vi "CRYUnflatten Post Processing.vi"(11 "Unflatten Post Processing":string) -> (0 "Error?":bool, 2 "Post-Processing":T1 {"user equation cluster"."Results axis" items=["x", "y", "z"]; "user equation cluster"."Input axis" items=["x", "y", "z"]; "user equation cluster"."Custom unit results array"."dB ref" format="%.2f"; "user equation cluster"."Custom unit input array"."dB ref" format="%.2f"; "Constant" format="%#.5p"; "Unary Operator" format="%10.0f"; "Custom unit info"."dB ref" format="%.2f"; "Sampling Rate" format="%#.2p"}, 3 "Header info":T3={"Data type"="Data            ", "Version"=1, "Dimensions"=0})   [LabVIEW 2013]
uses:
  Typedef Control/CRYPost Processing Cluster.ctl
  Typedef Control/CRYUser Equation Cluster.ctl
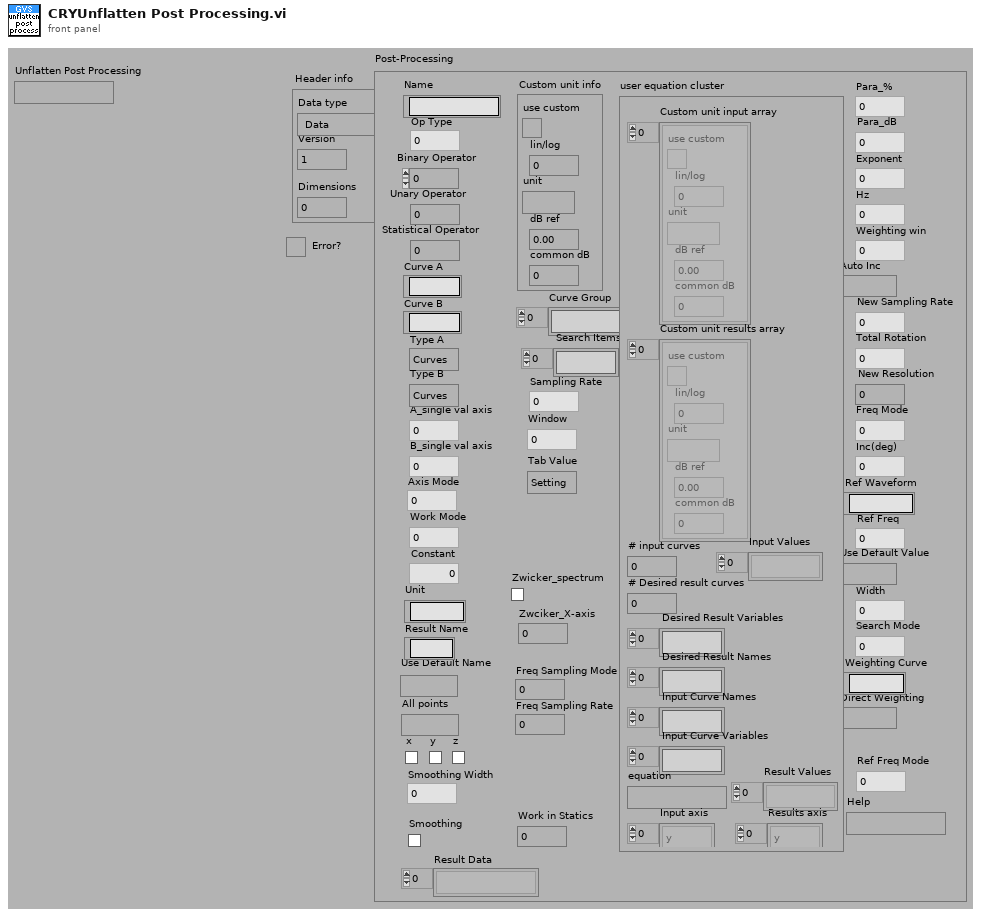
[diagram p1: front panel]
types:
  T1 = typedef "CRYPost Processing Cluster.ctl" = cluster{"Name":string, "Op Type":u16, "Curve A":string, "Curve B":string, "Axis Mode":u16, "Work Mode":u16, "Width":u16, "Weighting win":u16, "Search Mode":u16, "Freq Mode":u16, "New Sampling Rate":dbl, "Use Default Name":bool, "x":bool, "y":bool, "z":bool, "All points":bool, "A_single val axis":u16, "B_single val axis":u16, "Use Default Value":bool, "Result Name":string, "Smoothing Width":i32, "Window":u16, "Para_dB":sgl, "Para_%":sgl, "Exponent":sgl, "Hz":dbl, "Direct Weighting":bool, "Auto Inc":bool, "Inc(deg)":i32, "Total Rotation":i32, "Ref Freq Mode":u16, "Ref Waveform":string, "Sampling Rate":dbl, "Weighting Curve":string, "Ref Freq":dbl, "Curve Group":string[], "Search Items":string[], "Custom unit info":cluster{"use custom":bool, "lin/log":u16, "unit":string, "dB ref":dbl, "common dB":u16}, "Unit":string, "Type A":enum16{"Curves", "Values", "Results", "WFM"}, "Type B":enum16{"Curves", "Values", "Results", "WFM"}, "Unary Operator":u16, "Binary Operator":u16, "Statistical Operator":u16, "Constant ":dbl, "New Resolution":u16, "user equation cluster":T2, "Help":string, "Tab Value":enum32{"Setting", "Help"}, "Zwciker_X-axis":u16, "Zwicker_spectrum":bool, "Freq Sampling Mode":u16, "Freq Sampling Rate":dbl, "Smoothing":bool, "Work in Statics":u16, "Result Data":string[]}
  T2 = typedef "CRYUser Equation Cluster.ctl" = cluster{"Custom unit input array":cluster{"use custom":bool, "lin/log":u16, "unit":string, "dB ref":dbl, "common dB":u16}[], "Custom unit results array ":cluster{"use custom":bool, "lin/log":u16, "unit":string, "dB ref":dbl, "common dB":u16}[], "Desired Result Variables":string[], "Desired Result Names":string[], "Input Curve Names":string[], "Input Curve Variables":string[], "equation":string, "Input axis":u16[], "Results axis":u16[], "# input curves":i32, "# Desired result curves ":i32, "Input Values":string[], "Result Values":string[]}
  T3 = cluster{"Data type":string, "Version":u16, "Dimensions":u8}
  T4 = cluster{"Name":string, "Op Type":u16, "Curve A":string, "Curve B":string, "Axis Mode":u16, "Work Mode":u16, "Width":u16, "Weighting win":u16, "Search Mode":u16, "Freq Mode":u16, "New Sampling Rate":dbl, "Use Default Name":bool, "x":bool, "y":bool, "z":bool, "All points":bool, "A_single val axis":u16, "B_single val axis":u16, "Use Default Value":bool, "Result Name":string, "Smoothing Width":i32, "Window":u16, "Para_dB":sgl, "Para_%":sgl, "Exponent":sgl, "Hz":dbl, "Direct Weighting":bool, "Auto Inc":bool, "Inc(deg)":i32, "Total Rotation":i32, "Ref Freq Mode":u16, "Ref Waveform":string, "Sampling Rate":dbl, "Weighting Curve":string, "Ref Freq":dbl, "Curve Group":string[], "Search Items":string[], "Custom unit info":cluster{"use custom":bool, "lin/log":u16, "unit":string, "dB ref":dbl, "common dB":u16}, "Unit":string, "Type A":enum16{"Curves", "Values", "Results", "WFM"}, "Type B":enum16{"Curves", "Values", "Results", "WFM"}, "Unary Operator":u16, "Binary Operator":u16, "Statistical Operator":u16, "Constant ":dbl, "New Resolution":u16, "user equation cluster":T2, "Help":string, "Tab Value":enum32{"Setting", "Help"}, "Zwciker_X-axis":u16, "Zwicker_spectrum":bool, "Freq Sampling Mode":u16, "Freq Sampling Rate":dbl, "Smoothing":bool, "Work in Statics":u16, "Result Data":string[]}
  T5 = cluster{"unsigned byte array[0]":u8, "unsigned byte array[1]":u8, "unsigned byte array[2]":u8}
  T6 = cluster{"Name":string, "Op Type":u16, "Curve A":string, "Curve B":string, "Axis Mode":u16, "Work Mode":u16, "Width":u16, "Weighting win":u16, "Search Mode":u16, "Freq Mode":u16, "New Sampling Rate":dbl, "Use Default Name":bool, "x":bool, "y":bool, "z":bool, "All points":bool, "A_single val axis":u16, "B_single val axis":u16, "Use Default Value":bool, "Result Name":string, "Smoothing Width":i32, "Window":u16, "Para_dB":sgl, "Para_%":sgl, "Exponent":sgl, "Hz":u32, "Direct Weighting":bool, "Auto Inc":bool, "Inc(deg)":i32, "Total Rotation":i32, "Ref Freq Mode":u16, "Ref Waveform":string, "Sampling Rate":dbl, "Weighting Curve":string, "Ref Freq":dbl, "Curve Group":string[], "Search Items":string[], "Custom unit info":cluster{"use custom":bool, "lin/log":u16, "unit":string, "dB ref":dbl, "common dB":u16}, "Unit":string, "Type A":enum16{"Curves", "Values", "Results", "WFM"}, "Type B":enum16{"Curves", "Values", "Results", "WFM"}, "Unary Operator":u16, "Binary Operator":u16, "Statistical Operator":u16, "Constant ":dbl, "New Resolution":u16, "user equation cluster":T2}
  T7 = cluster{"use custom":bool, "lin/log":u16, "unit":string, "dB ref":dbl, "common dB":u16}
  T8 = cluster{"Name":string, "Op Type":u16, "Curve A":string, "Curve B":string, "Axis Mode":u16, "Work Mode":u16, "Width":u16, "Weighting win":u16, "Search Mode":u16, "Freq Mode":u16, "New Sampling Rate":dbl, "Use Default Name":bool, "x":bool, "y":bool, "z":bool, "All points":bool, "A_single val axis":u16, "B_single val axis":u16, "Use Default Value":bool, "Result Name":string, "Smoothing Width":i32, "Window":u16, "Para_dB":sgl, "Para_%":sgl, "Exponent":sgl, "Hz":u32, "Direct Weighting":bool, "Auto Inc":bool, "Inc(deg)":i32, "Total Rotation":i32, "Ref Freq Mode":u16, "Ref Waveform":string, "Sampling Rate":dbl, "Weighting Curve":string, "Ref Freq":dbl, "Curve Group":string[], "Search Items":string[], "Custom unit info":cluster{"use custom":bool, "lin/log":u16, "unit":string, "dB ref":dbl, "common dB":u16}, "Unit":string, "Type A":enum16{"Curves", "Values", "Results", "WFM"}, "Type B":enum16{"Curves", "Values", "Results", "WFM"}, "Unary Operator":u16, "Binary Operator":u16, "Statistical Operator":u16, "Constant ":dbl, "New Resolution":u16, "user equation cluster":T2, "Help":string, "Tab Value":enum32{"Setting", "Help"}}
  T9 = cluster{"Name":string, "Op Type":u16, "Curve A":string, "Curve B":string, "Axis Mode":u16, "Work Mode":u16, "Width":u16, "Weighting win":u16, "Search Mode":u16, "Freq Mode":u16, "New Sampling Rate":dbl, "Use Default Name":bool, "x":bool, "y":bool, "z":bool, "All points":bool, "A_single val axis":u16, "B_single val axis":u16, "Use Default Value":bool, "Result Name":string, "Smoothing Width":i32, "Window":u16, "Para_dB":sgl, "Para_%":sgl, "Exponent":sgl, "Hz":dbl, "Direct Weighting":bool, "Auto Inc":bool, "Inc(deg)":i32, "Total Rotation":i32, "Ref Freq Mode":u16, "Ref Waveform":string, "Sampling Rate":dbl, "Weighting Curve":string, "Ref Freq":dbl, "Curve Group":string[], "Search Items":string[], "Custom unit info":cluster{"use custom":bool, "lin/log":u16, "unit":string, "dB ref":dbl, "common dB":u16}, "Unit":string, "Type A":enum16{"Curves", "Values", "Results", "WFM"}, "Type B":enum16{"Curves", "Values", "Results", "WFM"}, "Unary Operator":u16, "Binary Operator":u16, "Statistical Operator":u16, "Constant ":dbl, "New Resolution":u16, "user equation cluster":T2, "Help":string, "Tab Value":enum32{"Setting", "Help"}}
  T10 = cluster{"Name":string, "Op Type":u16, "Curve A":string, "Curve B":string, "Axis Mode":u16, "Work Mode":u16, "Width":u16, "Weighting win":u16, "Search Mode":u16, "Freq Mode":u16, "New Sampling Rate":dbl, "Use Default Name":bool, "x":bool, "y":bool, "z":bool, "All points":bool, "A_single val axis":u16, "B_single val axis":u16, "Use Default Value":bool, "Result Name":string, "Smoothing Width":i32, "Window":u16, "Para_dB":sgl, "Para_%":sgl, "Exponent":sgl, "Hz":dbl, "Direct Weighting":bool, "Auto Inc":bool, "Inc(deg)":i32, "Total Rotation":i32, "Ref Freq Mode":u16, "Ref Waveform":string, "Sampling Rate":dbl, "Weighting Curve":string, "Ref Freq":dbl, "Curve Group":string[], "Search Items":string[], "Custom unit info":cluster{"use custom":bool, "lin/log":u16, "unit":string, "dB ref":dbl, "common dB":u16}, "Unit":string, "Type A":enum16{"Curves", "Values", "Results", "WFM"}, "Type B":enum16{"Curves", "Values", "Results", "WFM"}, "Unary Operator":u16, "Binary Operator":u16, "Statistical Operator":u16, "Constant ":dbl, "New Resolution":u16, "user equation cluster":T2, "Help":string, "Tab Value":enum32{"Setting", "Help"}, "Zwciker_X-axis":u16, "Zwicker_spectrum":bool}
  T11 = cluster{"Name":string, "Op Type":u16, "Curve A":string, "Curve B":string, "Axis Mode":u16, "Work Mode":u16, "Width":u16, "Weighting win":u16, "Search Mode":u16, "Freq Mode":u16, "New Sampling Rate":dbl, "Use Default Name":bool, "x":bool, "y":bool, "z":bool, "All points":bool, "A_single val axis":u16, "B_single val axis":u16, "Use Default Value":bool, "Result Name":string, "Smoothing Width":i32, "Window":u16, "Para_dB":sgl, "Para_%":sgl, "Exponent":sgl, "Hz":dbl, "Direct Weighting":bool, "Auto Inc":bool, "Inc(deg)":i32, "Total Rotation":i32, "Ref Freq Mode":u16, "Ref Waveform":string, "Sampling Rate":dbl, "Weighting Curve":string, "Ref Freq":dbl, "Curve Group":string[], "Search Items":string[], "Custom unit info":cluster{"use custom":bool, "lin/log":u16, "unit":string, "dB ref":dbl, "common dB":u16}, "Unit":string, "Type A":enum16{"Curves", "Values", "Results", "WFM"}, "Type B":enum16{"Curves", "Values", "Results", "WFM"}, "Unary Operator":u16, "Binary Operator":u16, "Statistical Operator":u16, "Constant ":dbl, "New Resolution":u16, "user equation cluster":T2, "Help":string, "Tab Value":enum32{"Setting", "Help"}, "Zwciker_X-axis":u16, "Zwicker_spectrum":bool, "Freq Sampling Mode":u16, "Freq Sampling Rate":dbl}
  T12 = cluster{"Name":string, "Op Type":u16, "Curve A":string, "Curve B":string, "Axis Mode":u16, "Work Mode":u16, "Width":u16, "Weighting win":u16, "Search Mode":u16, "Freq Mode":u16, "New Sampling Rate":dbl, "Use Default Name":bool, "x":bool, "y":bool, "z":bool, "All points":bool, "A_single val axis":u16, "B_single val axis":u16, "Use Default Value":bool, "Result Name":string, "Smoothing Width":i32, "Window":u16, "Para_dB":sgl, "Para_%":sgl, "Exponent":sgl, "Hz":dbl, "Direct Weighting":bool, "Auto Inc":bool, "Inc(deg)":i32, "Total Rotation":i32, "Ref Freq Mode":u16, "Ref Waveform":string, "Sampling Rate":dbl, "Weighting Curve":string, "Ref Freq":dbl, "Curve Group":string[], "Search Items":string[], "Custom unit info":cluster{"use custom":bool, "lin/log":u16, "unit":string, "dB ref":dbl, "common dB":u16}, "Unit":string, "Type A":enum16{"Curves", "Values", "Results", "WFM"}, "Type B":enum16{"Curves", "Values", "Results", "WFM"}, "Unary Operator":u16, "Binary Operator":u16, "Statistical Operator":u16, "Constant ":dbl, "New Resolution":u16, "user equation cluster":T2, "Help":string, "Tab Value":enum32{"Setting", "Help"}, "Zwciker_X-axis":u16, "Zwicker_spectrum":bool, "Freq Sampling Mode":u16, "Freq Sampling Rate":dbl, "Smoothing":bool}
  T13 = cluster{"Name":string, "Op Type":u16, "Curve A":string, "Curve B":string, "Axis Mode":u16, "Work Mode":u16, "Width":u16, "Weighting win":u16, "Search Mode":u16, "Freq Mode":u16, "New Sampling Rate":dbl, "Use Default Name":bool, "x":bool, "y":bool, "z":bool, "All points":bool, "A_single val axis":u16, "B_single val axis":u16, "Use Default Value":bool, "Result Name":string, "Smoothing Width":i32, "Window":u16, "Para_dB":sgl, "Para_%":sgl, "Exponent":sgl, "Hz":dbl, "Direct Weighting":bool, "Auto Inc":bool, "Inc(deg)":i32, "Total Rotation":i32, "Ref Freq Mode":u16, "Ref Waveform":string, "Sampling Rate":dbl, "Weighting Curve":string, "Ref Freq":dbl, "Curve Group":string[], "Search Items":string[], "Custom unit info":cluster{"use custom":bool, "lin/log":u16, "unit":string, "dB ref":dbl, "common dB":u16}, "Unit":string, "Type A":enum16{"Curves", "Values", "Results", "WFM"}, "Type B":enum16{"Curves", "Values", "Results", "WFM"}, "Unary Operator":u16, "Binary Operator":u16, "Statistical Operator":u16, "Constant ":dbl, "New Resolution":u16, "user equation cluster":T2, "Help":string, "Tab Value":enum32{"Setting", "Help"}, "Zwciker_X-axis":u16, "Zwicker_spectrum":bool, "Freq Sampling Mode":u16, "Freq Sampling Rate":dbl, "Smoothing":bool, "Work in Statics":u16}
  T14 = cluster{"substring":string, u16, "unsigned byte array[2]":u8}
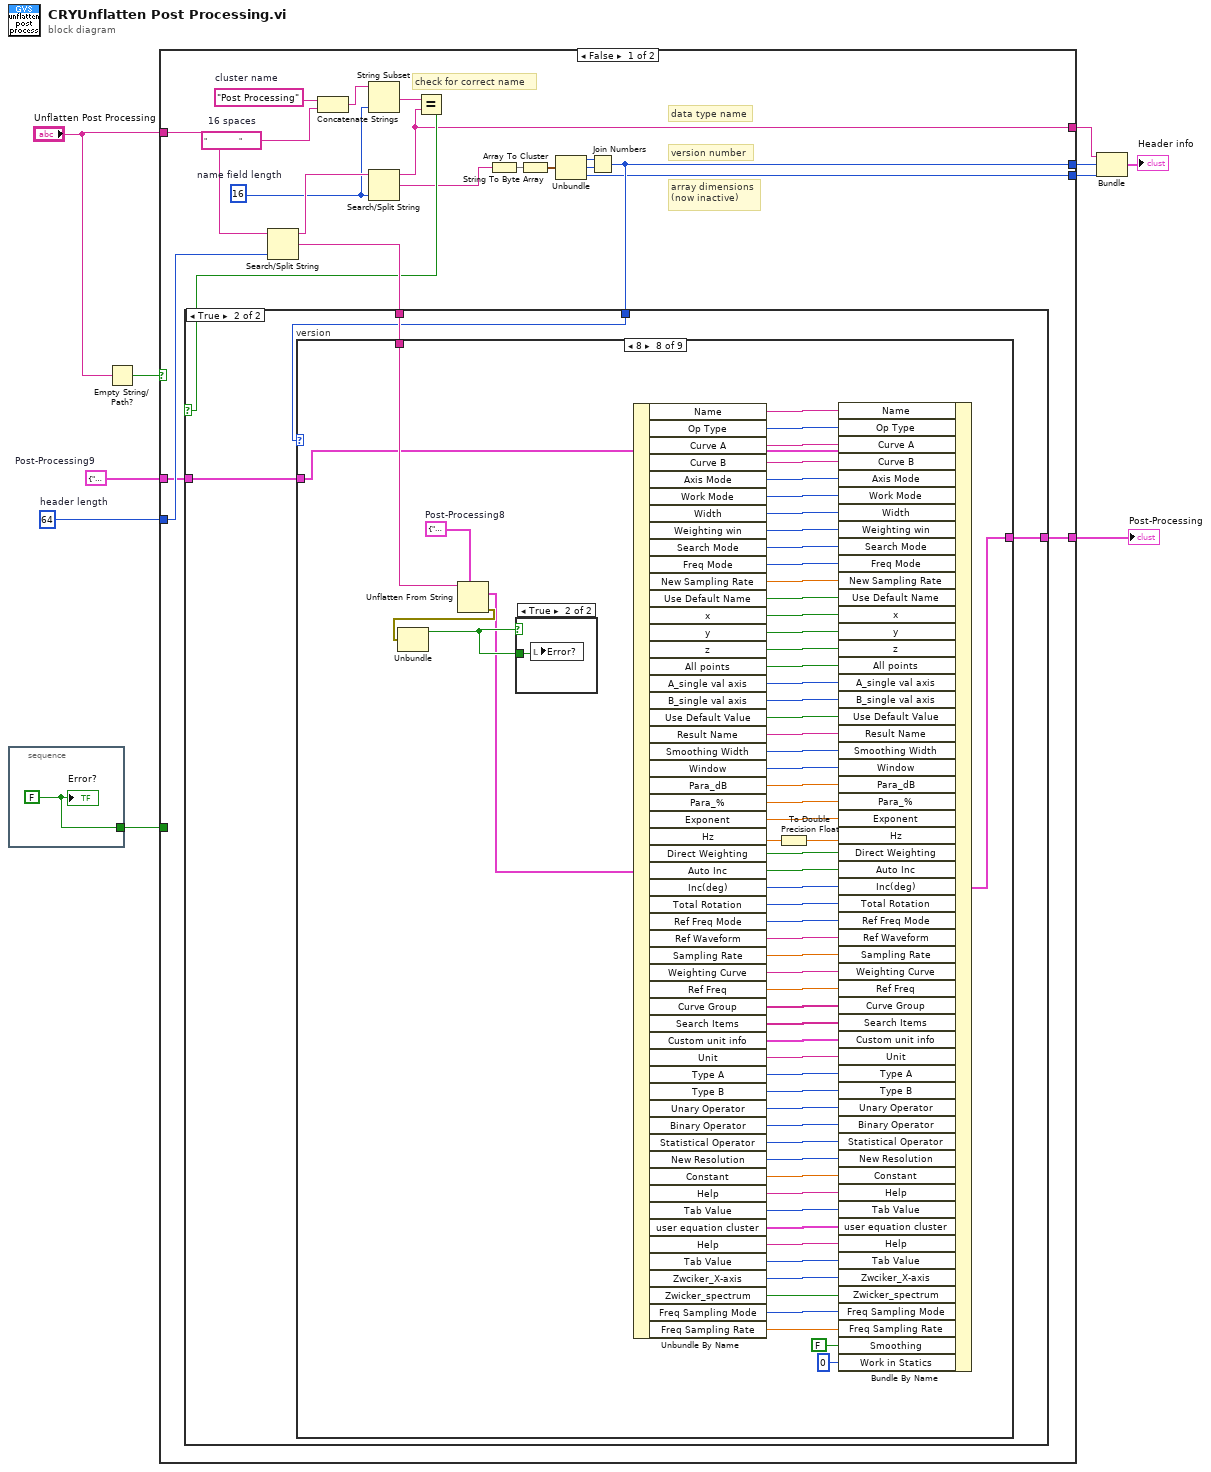
[diagram p0: block diagram]
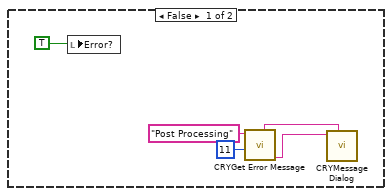
[diagram p2: hidden frame]
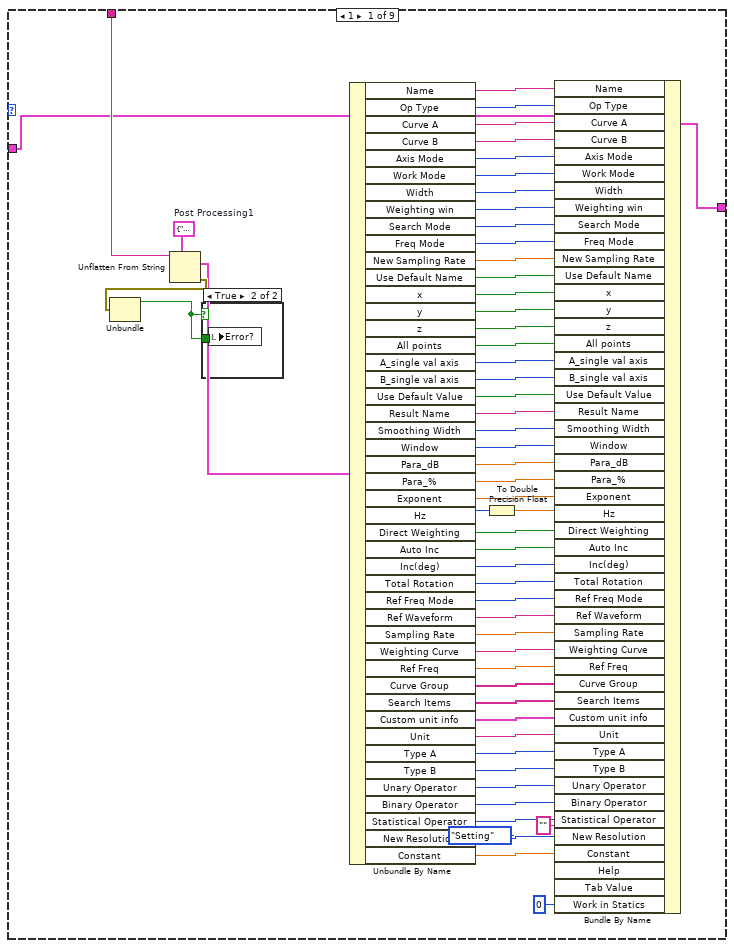
[diagram p3: hidden frame]
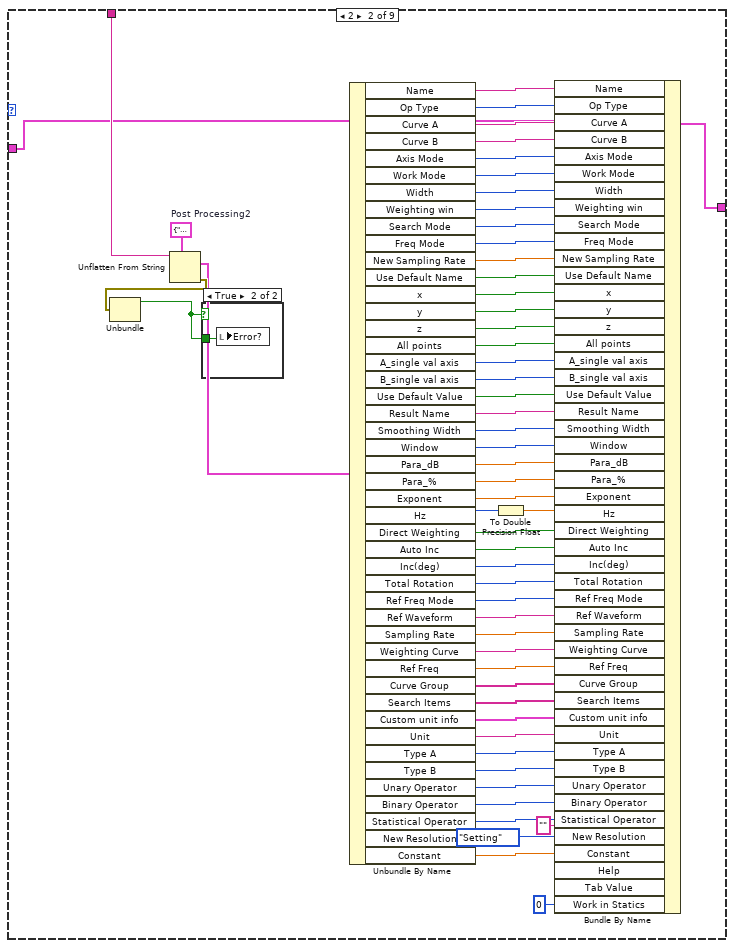
[diagram p5: hidden frame]
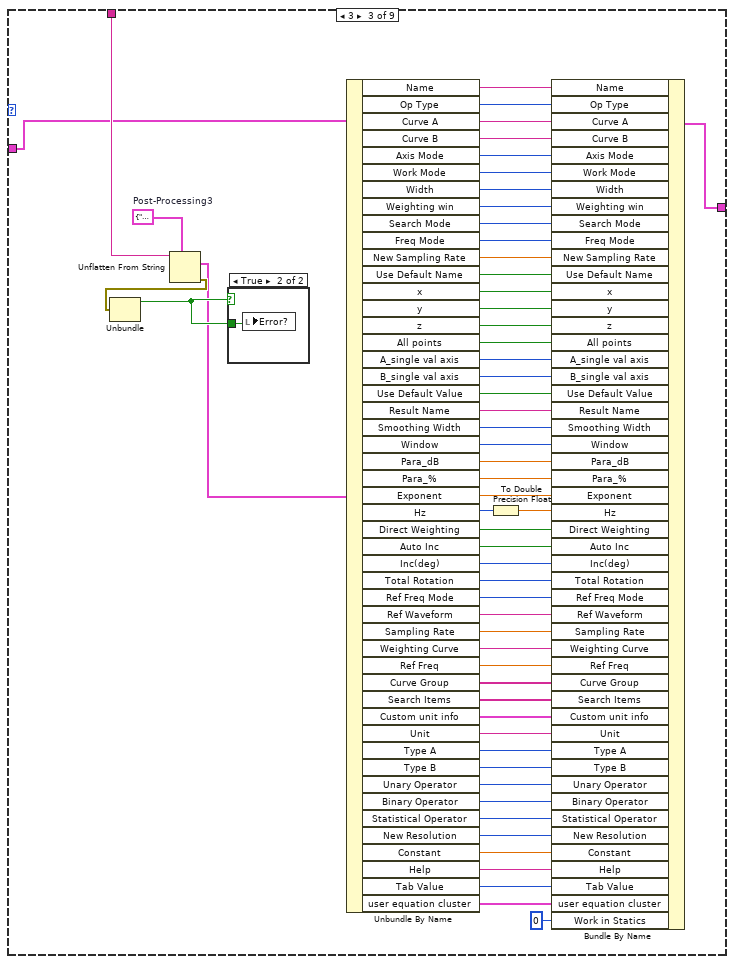
[diagram p7: hidden frame]
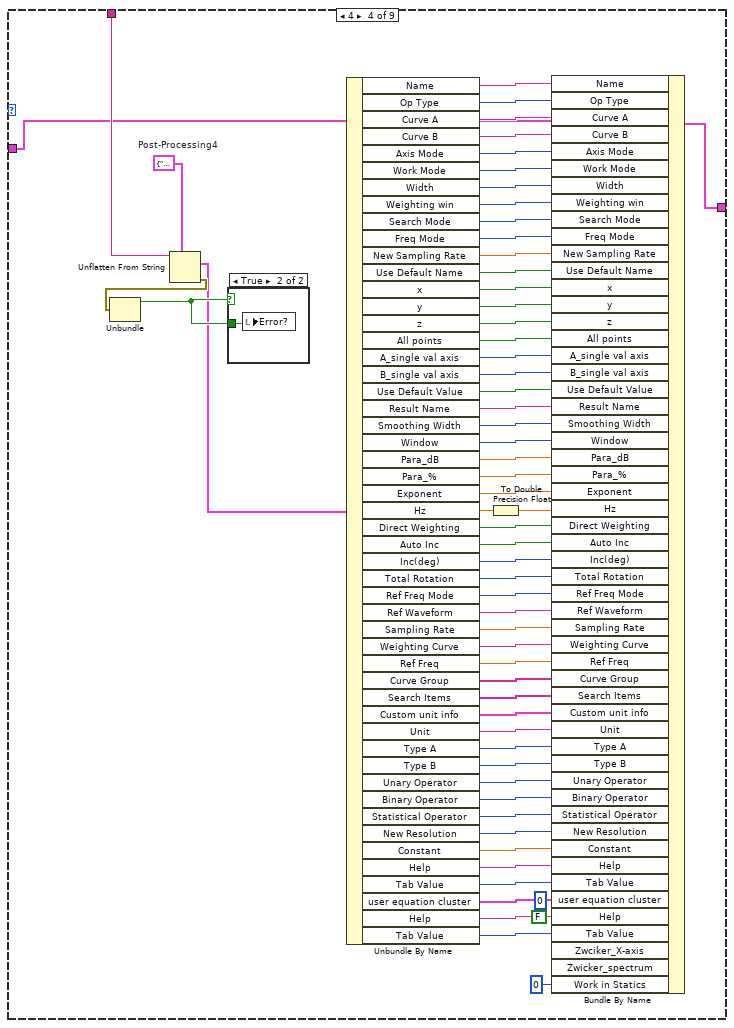
[diagram p9: hidden frame]
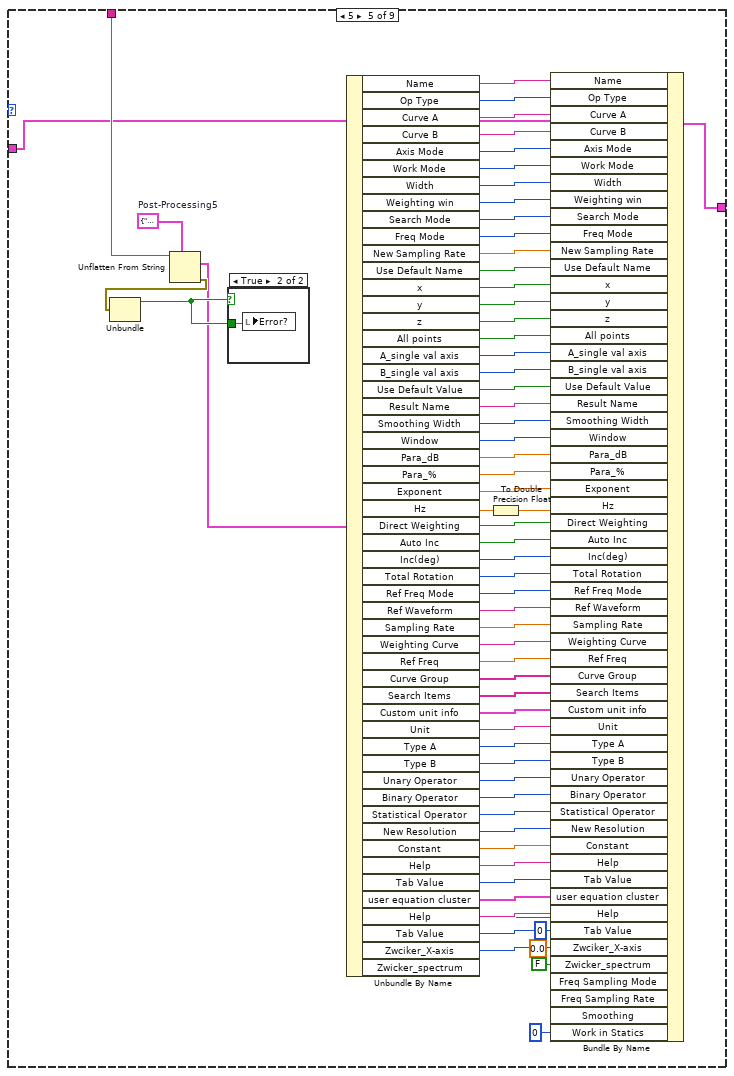
[diagram p11: hidden frame]
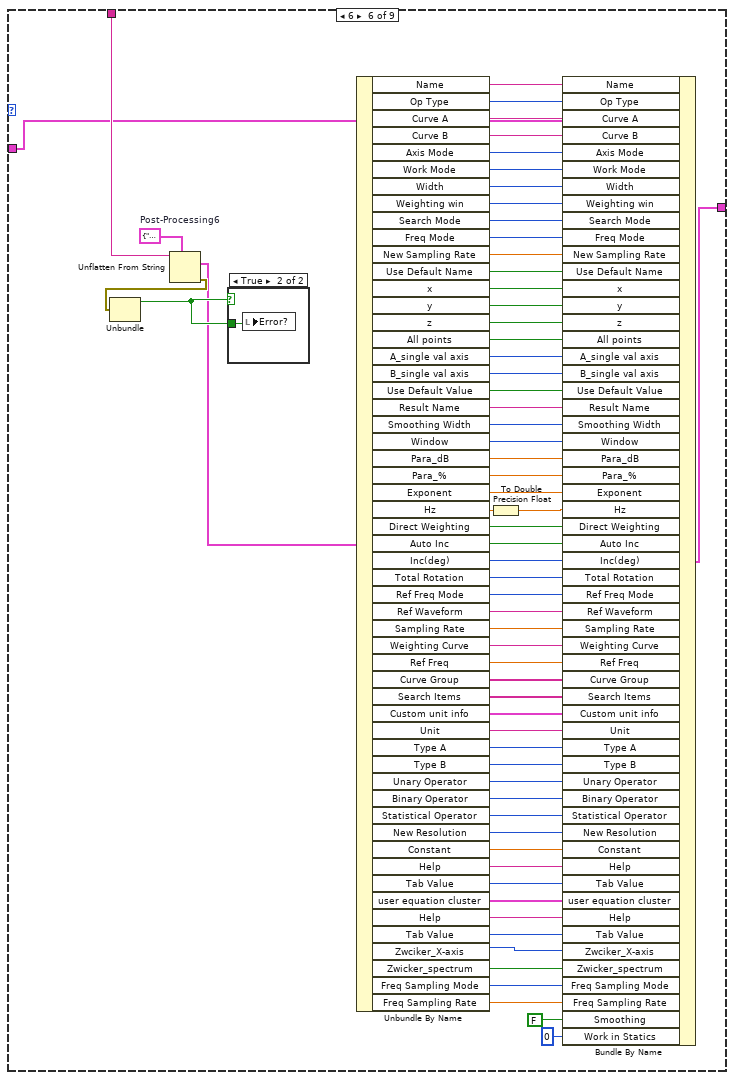
[diagram p13: hidden frame]
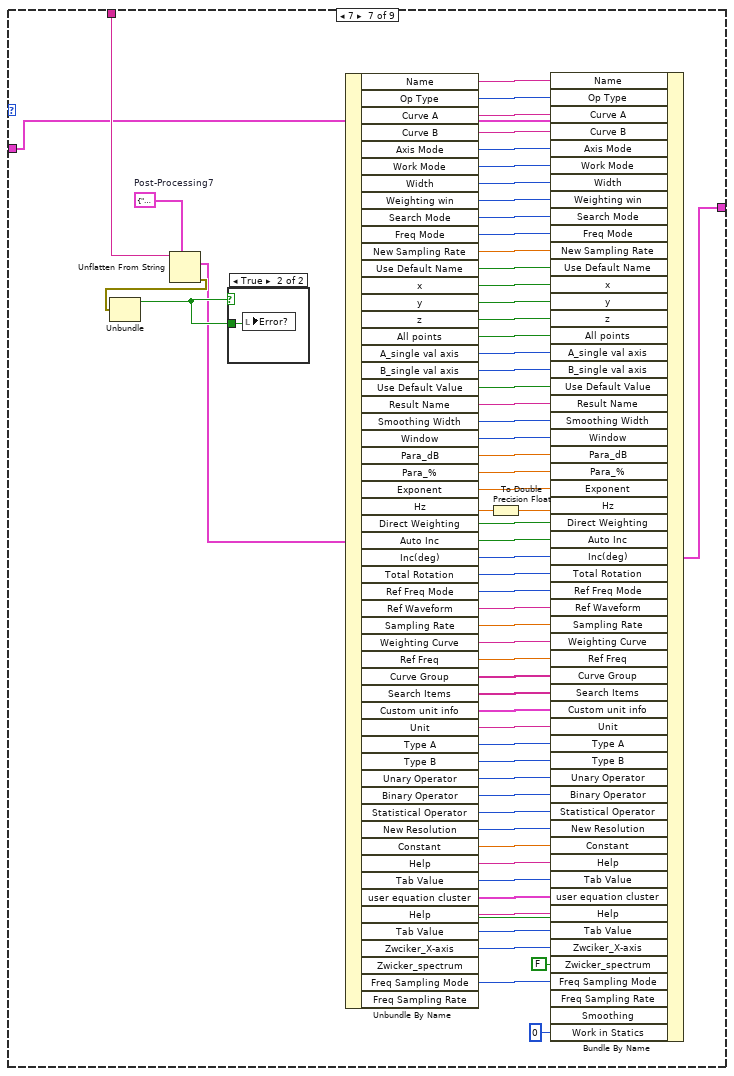
[diagram p15: hidden frame]
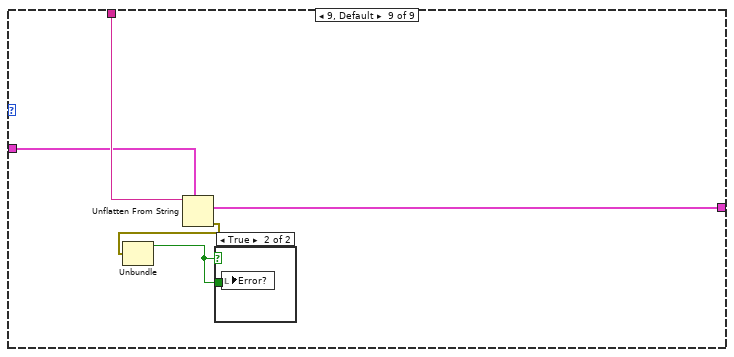
[diagram p18: hidden frame]
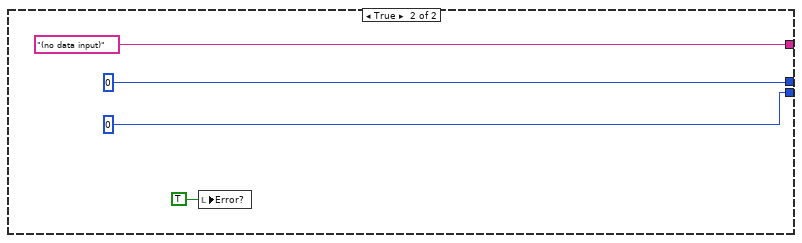
[diagram p20: hidden frame]
diagram:
  w2 = T4 {"Name"="", "Op Type"=0, "Curve A"="", "Curve B"="", "Axis Mode"=0, "Work Mode"=0, "Width"=0, "Weighting win"=0, "Search Mode"=0, "Freq Mode"=0, "New Sampling Rate"=0.0, "Use Default Name"=FALSE, "x"=FALSE, "y"=FALSE, "z"=FALSE, "All points"=FALSE, "A_single val axis"=0, "B_single val axis"=0, "Use Default Value"=FALSE, "Result Name"="", "Smoothing Width"=0, "Window"=0, "Para_dB"=0.0, "Para_%"=0.0, "Exponent"=0.0, "Hz"=0.0, "Direct Weighting"=FALSE, "Auto Inc"=FALSE, "Inc(deg)"=0, "Total Rotation"=0, "Ref Freq Mode"=0, "Ref Waveform"="", "Sampling Rate"=0.0, "Weighting Curve"="", "Ref Freq"=0.0, "Curve Group"=[], "Search Items"=[], "Custom unit info"={"use custom"=FALSE, "lin/log"=0, "unit"="", "dB ref"=0.0, "common dB"=0}, "Unit"="", "Type A"=enum."Curves", "Type B"=enum."Curves", "Unary Operator"=0, "Binary Operator"=0, "Statistical Operator"=0, "Constant "=0.0, "New Resolution"=0, "user equation cluster"={"Custom unit input array"=[], "Custom unit results array "=[], "Desired Result Variables"=[], "Desired Result Names"=[], "Input Curve Names"=[], "Input Curve Variables"=[], "equation"="", "Input axis"=[], "Results axis"=[], "# input curves"=0, "# Desired result curves "=0, "Input Values"=[], "Result Values"=[]}, "Help"="", "Tab Value"=enum."Setting", "Zwciker_X-axis"=0, "Zwicker_spectrum"=FALSE, "Freq Sampling Mode"=0, "Freq Sampling Rate"=0.0, "Smoothing"=FALSE, "Work in Statics"=0, "Result Data"=[]}  # Post-Processing9
  w8 = 64  # header length
  n1 = stacked-sequence {
    tunnel: [w11] -> w3
    frame #0 {
      w11 = FALSE
      "Error?" <- w11
    }
  }
  n2 = Empty String/Path?(string/path="Unflatten Post Processing") -> (empty?=w9:bool)
  n3 = case shown="False" w9 {
    tunnel: "Unflatten Post Processing" -> [w31 _]
    tunnel: w8 -> [w25 _]
    tunnel: [w22 u16 0] -> w6
    tunnel: [w14 u8 0] -> w7
    tunnel: [w15 "(no data input)" ("substring")] -> w5
    tunnel: w3 -> [_ _]
    tunnel: [w13 _] -> w1
    tunnel: w2 -> [w12 _]
    frame False {
      w19 = "                "  # 16 spaces
      w20 = "Post Processing"  # cluster name
      w17 = 16  # name field length
      # "check for correct name"
      # "array dimensions\n(now inactive)"
      # "version number"
      # "data type name"
      n4 = Search/Split String(string=w31, offset (0)=w25) -> (substring before match=w24:string, match + rest of string=w26:string)  [unwired: 2 out]
      n5 = Concatenate Strings(w20, w19) -> (w18:string)
      n6 = String Subset(string=w18, length (rest)=w17) -> (substring=w16:string)  [unwired: 1 out]
      n7 = Search/Split String(string=w24, offset (0)=w17) -> (substring before match=w15:string, match + rest of string=w21:string)  [unwired: 2 out]
      n8 = Equal?(x=w16, y=w15) -> (x = y?=w23:bool)
      n9 = String To Byte Array(string=w21) -> (unsigned byte array=w30:u8[])
      n10 = Array To Cluster(array=w30) -> (cluster=w29:T5)
      n11 = Unbundle(w29) -> ("unsigned byte array[0]"=w28:u8, "unsigned byte array[1]"=w27:u8, "unsigned byte array[2]"=w14:u8)
      n12 = Join Numbers(hi=w28, lo=w27) -> ((hi.lo)=w22:u16)
      n13 = case shown="True" w23 {
        tunnel: w26 -> [_ w40]
        tunnel: w22 -> [_ w39]
        tunnel: [_ w38] -> w13
        tunnel: w12 -> [_ w37]
        frame False {
          n14 = local write "Error?"(TRUE) -> ()
          n15 = call "CRYGet Error Message.vi"("Error No"=11 ("No"), "Kind"="Post Processing") -> ("Message Sub 3"=w32:string, "Window Title"=w33:string)  [unwired: 4 in, 4 out]
          n16 = call "CRYMessage Dialog.vi"("Window Title"=w33, "Message Content"=w32) -> ()  [unwired: 8 in, 2 out]
        }
        frame True {
          n17 = case "version" shown="8" w39 {
            tunnel: w40 -> [w97 w155 w214 w277 w343 w409 w475 w541 w545]
            tunnel: [w92 w150 w210 w273 w339 w405 w471 w537 w544] -> w38
            tunnel: w37 -> [w45 w103 w163 w226 w292 w358 w424 w490 w543]
            frame 1 {
              w94 = T6 {"Name"="", "Op Type"=0, "Curve A"="", "Curve B"="", "Axis Mode"=0, "Work Mode"=0, "Width"=0, "Weighting win"=0, "Search Mode"=0, "Freq Mode"=0, "New Sampling Rate"=0.0, "Use Default Name"=FALSE, "x"=FALSE, "y"=FALSE, "z"=FALSE, "All points"=FALSE, "A_single val axis"=0, "B_single val axis"=0, "Use Default Value"=FALSE, "Result Name"="", "Smoothing Width"=0, "Window"=0, "Para_dB"=0.0, "Para_%"=0.0, "Exponent"=0.0, "Hz"=0, "Direct Weighting"=FALSE, "Auto Inc"=FALSE, "Inc(deg)"=0, "Total Rotation"=0, "Ref Freq Mode"=0, "Ref Waveform"="", "Sampling Rate"=0.0, "Weighting Curve"="", "Ref Freq"=0.0, "Curve Group"=[], "Search Items"=[], "Custom unit info"={"use custom"=FALSE, "lin/log"=0, "unit"="", "dB ref"=0.0, "common dB"=0}, "Unit"="", "Type A"=enum."Curves", "Type B"=enum."Curves", "Unary Operator"=0, "Binary Operator"=0, "Statistical Operator"=0, "Constant "=0.0, "New Resolution"=0, "user equation cluster"={"Custom unit input array"=[], "Custom unit results array "=[], "Desired Result Variables"=[], "Desired Result Names"=[], "Input Curve Names"=[], "Input Curve Variables"=[], "equation"="", "Input axis"=[], "Results axis"=[], "# input curves"=0, "# Desired result curves "=0, "Input Values"=[], "Result Values"=[]}}  # Post Processing1
              n18 = Unflatten From String(type=w94, binary string=w97) -> (value=w93:T6, error out=w95:errorcluster)  [unwired: 1 in, 3 out]
              n19 = Unbundle(w95) -> ("status"=w96:bool)  [unwired: 2 out]
              n20 = case shown="True" w96 {
                tunnel: w96 -> [_ w98]
                frame False {
                }
                frame True {
                  n21 = local write "Error?"(w98) -> ()
                }
              }
              n22 = Unbundle By Name(w93) -> ("Name"=w91:string, "Op Type"=w90:u16, "Curve A"=w89:string, "Curve B"=w88:string, "Axis Mode"=w87:u16, "Work Mode"=w86:u16, "Width"=w85:u16, "Weighting win"=w84:u16, "Search Mode"=w83:u16, "Freq Mode"=w82:u16, "New Sampling Rate"=w81:dbl, "Use Default Name"=w80:bool, "x"=w79:bool, "y"=w78:bool, "z"=w77:bool, "All points"=w76:bool, "A_single val axis"=w75:u16, "B_single val axis"=w74:u16, "Use Default Value"=w73:bool, "Result Name"=w72:string, "Smoothing Width"=w71:i32, "Window"=w70:u16, "Para_dB"=w69:sgl, "Para_%"=w68:sgl, "Exponent"=w67:sgl, "Hz"=w66:u32, "Direct Weighting"=w65:bool, "Auto Inc"=w64:bool, "Inc(deg)"=w63:i32, "Total Rotation"=w62:i32, "Ref Freq Mode"=w61:u16, "Ref Waveform"=w60:string, "Sampling Rate"=w59:dbl, "Weighting Curve"=w58:string, "Ref Freq"=w57:dbl, "Curve Group"=w56:string[], "Search Items"=w55:string[], "Custom unit info"=w54:T7, "Unit"=w53:string, "Type A"=w52:enum16{"Curves", "Values", "Results", "WFM"}, "Type B"=w51:enum16{"Curves", "Values", "Results", "WFM"}, "Unary Operator"=w50:u16, "Binary Operator"=w49:u16, "Statistical Operator"=w48:u16, "New Resolution"=w47:u16, "Constant"=w46:dbl)
              n23 = To Double Precision Float(number=w66) -> (double precision float=w42:dbl)
              n24 = Bundle By Name(cluster=w45, "Name"=w91, "Op Type"=w90, "Curve A"=w89, "Curve B"=w88, "Axis Mode"=w87, "Work Mode"=w86, "Width"=w85, "Weighting win"=w84, "Search Mode"=w83, "Freq Mode"=w82, "New Sampling Rate"=w81, "Use Default Name"=w80, "x"=w79, "y"=w78, "z"=w77, "All points"=w76, "A_single val axis"=w75, "B_single val axis"=w74, "Use Default Value"=w73, "Result Name"=w72, "Smoothing Width"=w71, "Window"=w70, "Para_dB"=w69, "Para_%"=w68, "Exponent"=w67, "Hz"=w42, "Direct Weighting"=w65, "Auto Inc"=w64, "Inc(deg)"=w63, "Total Rotation"=w62, "Ref Freq Mode"=w61, "Ref Waveform"=w60, "Sampling Rate"=w59, "Weighting Curve"=w58, "Ref Freq"=w57, "Curve Group"=w56, "Search Items"=w55, "Custom unit info"=w54, "Unit"=w53, "Type A"=w52, "Type B"=w51, "Unary Operator"=w50, "Binary Operator"=w49, "Statistical Operator"=w48, "New Resolution"=w47, "Constant"=w46, "Help"="", "Tab Value"=enum32{"Setting", "Help"}."Setting", "Work in Statics"=u16 0) -> (w92:T4)
            }
            frame 2 {
              w152 = T6 {"Name"="", "Op Type"=0, "Curve A"="", "Curve B"="", "Axis Mode"=0, "Work Mode"=0, "Width"=0, "Weighting win"=0, "Search Mode"=0, "Freq Mode"=0, "New Sampling Rate"=0.0, "Use Default Name"=FALSE, "x"=FALSE, "y"=FALSE, "z"=FALSE, "All points"=FALSE, "A_single val axis"=0, "B_single val axis"=0, "Use Default Value"=FALSE, "Result Name"="", "Smoothing Width"=0, "Window"=0, "Para_dB"=0.0, "Para_%"=0.0, "Exponent"=0.0, "Hz"=0, "Direct Weighting"=FALSE, "Auto Inc"=FALSE, "Inc(deg)"=0, "Total Rotation"=0, "Ref Freq Mode"=0, "Ref Waveform"="", "Sampling Rate"=0.0, "Weighting Curve"="", "Ref Freq"=0.0, "Curve Group"=[], "Search Items"=[], "Custom unit info"={"use custom"=FALSE, "lin/log"=0, "unit"="", "dB ref"=0.0, "common dB"=0}, "Unit"="", "Type A"=enum."Curves", "Type B"=enum."Curves", "Unary Operator"=0, "Binary Operator"=0, "Statistical Operator"=0, "Constant "=0.0, "New Resolution"=0, "user equation cluster"={"Custom unit input array"=[], "Custom unit results array "=[], "Desired Result Variables"=[], "Desired Result Names"=[], "Input Curve Names"=[], "Input Curve Variables"=[], "equation"="", "Input axis"=[], "Results axis"=[], "# input curves"=0, "# Desired result curves "=0, "Input Values"=[], "Result Values"=[]}}  # Post Processing2
              n25 = Unflatten From String(type=w152, binary string=w155) -> (value=w151:T6, error out=w153:errorcluster)  [unwired: 1 in, 3 out]
              n26 = Unbundle(w153) -> ("status"=w154:bool)  [unwired: 2 out]
              n27 = case shown="True" w154 {
                tunnel: w154 -> [_ w156]
                frame False {
                }
                frame True {
                  n28 = local write "Error?"(w156) -> ()
                }
              }
              n29 = Unbundle By Name(w151) -> ("Name"=w149:string, "Op Type"=w148:u16, "Curve A"=w147:string, "Curve B"=w146:string, "Axis Mode"=w145:u16, "Work Mode"=w144:u16, "Width"=w143:u16, "Weighting win"=w142:u16, "Search Mode"=w141:u16, "Freq Mode"=w140:u16, "New Sampling Rate"=w139:dbl, "Use Default Name"=w138:bool, "x"=w137:bool, "y"=w136:bool, "z"=w135:bool, "All points"=w134:bool, "A_single val axis"=w133:u16, "B_single val axis"=w132:u16, "Use Default Value"=w131:bool, "Result Name"=w130:string, "Smoothing Width"=w129:i32, "Window"=w128:u16, "Para_dB"=w127:sgl, "Para_%"=w126:sgl, "Exponent"=w125:sgl, "Hz"=w124:u32, "Direct Weighting"=w123:bool, "Auto Inc"=w122:bool, "Inc(deg)"=w121:i32, "Total Rotation"=w120:i32, "Ref Freq Mode"=w119:u16, "Ref Waveform"=w118:string, "Sampling Rate"=w117:dbl, "Weighting Curve"=w116:string, "Ref Freq"=w115:dbl, "Curve Group"=w114:string[], "Search Items"=w113:string[], "Custom unit info"=w112:T7, "Unit"=w111:string, "Type A"=w110:enum16{"Curves", "Values", "Results", "WFM"}, "Type B"=w109:enum16{"Curves", "Values", "Results", "WFM"}, "Unary Operator"=w108:u16, "Binary Operator"=w107:u16, "Statistical Operator"=w106:u16, "New Resolution"=w105:u16, "Constant"=w104:dbl)
              n30 = To Double Precision Float(number=w124) -> (double precision float=w100:dbl)
              n31 = Bundle By Name(cluster=w103, "Name"=w149, "Op Type"=w148, "Curve A"=w147, "Curve B"=w146, "Axis Mode"=w145, "Work Mode"=w144, "Width"=w143, "Weighting win"=w142, "Search Mode"=w141, "Freq Mode"=w140, "New Sampling Rate"=w139, "Use Default Name"=w138, "x"=w137, "y"=w136, "z"=w135, "All points"=w134, "A_single val axis"=w133, "B_single val axis"=w132, "Use Default Value"=w131, "Result Name"=w130, "Smoothing Width"=w129, "Window"=w128, "Para_dB"=w127, "Para_%"=w126, "Exponent"=w125, "Hz"=w100, "Direct Weighting"=w123, "Auto Inc"=w122, "Inc(deg)"=w121, "Total Rotation"=w120, "Ref Freq Mode"=w119, "Ref Waveform"=w118, "Sampling Rate"=w117, "Weighting Curve"=w116, "Ref Freq"=w115, "Curve Group"=w114, "Search Items"=w113, "Custom unit info"=w112, "Unit"=w111, "Type A"=w110, "Type B"=w109, "Unary Operator"=w108, "Binary Operator"=w107, "Statistical Operator"=w106, "New Resolution"=w105, "Constant"=w104, "Help"="", "Tab Value"=enum32{"Setting", "Help"}."Setting", "Work in Statics"=u16 0) -> (w150:T4)
            }
            frame 3 {
              w161 = T8 {"Name"="", "Op Type"=0, "Curve A"="", "Curve B"="", "Axis Mode"=0, "Work Mode"=0, "Width"=0, "Weighting win"=0, "Search Mode"=0, "Freq Mode"=0, "New Sampling Rate"=0.0, "Use Default Name"=FALSE, "x"=FALSE, "y"=FALSE, "z"=FALSE, "All points"=FALSE, "A_single val axis"=0, "B_single val axis"=0, "Use Default Value"=FALSE, "Result Name"="", "Smoothing Width"=0, "Window"=0, "Para_dB"=0.0, "Para_%"=0.0, "Exponent"=0.0, "Hz"=0, "Direct Weighting"=FALSE, "Auto Inc"=FALSE, "Inc(deg)"=0, "Total Rotation"=0, "Ref Freq Mode"=0, "Ref Waveform"="", "Sampling Rate"=0.0, "Weighting Curve"="", "Ref Freq"=0.0, "Curve Group"=[], "Search Items"=[], "Custom unit info"={"use custom"=FALSE, "lin/log"=0, "unit"="", "dB ref"=0.0, "common dB"=0}, "Unit"="", "Type A"=enum."Curves", "Type B"=enum."Curves", "Unary Operator"=0, "Binary Operator"=0, "Statistical Operator"=0, "Constant "=0.0, "New Resolution"=0, "user equation cluster"={"Custom unit input array"=[], "Custom unit results array "=[], "Desired Result Variables"=[], "Desired Result Names"=[], "Input Curve Names"=[], "Input Curve Variables"=[], "equation"="", "Input axis"=[], "Results axis"=[], "# input curves"=0, "# Desired result curves "=0, "Input Values"=[], "Result Values"=[]}, "Help"="", "Tab Value"=enum."Setting"}  # Post-Processing3
              n32 = Unflatten From String(type=w161, binary string=w214) -> (value=w211:T8, error out=w212:errorcluster)  [unwired: 1 in, 3 out]
              n33 = Unbundle(w212) -> ("status"=w213:bool)  [unwired: 2 out]
              n34 = case shown="True" w213 {
                tunnel: w213 -> [_ w215]
                frame False {
                }
                frame True {
                  n35 = local write "Error?"(w215) -> ()
                }
              }
              n36 = Unbundle By Name(w211) -> ("Name"=w209:string, "Op Type"=w208:u16, "Curve A"=w207:string, "Curve B"=w206:string, "Axis Mode"=w205:u16, "Work Mode"=w204:u16, "Width"=w203:u16, "Weighting win"=w202:u16, "Search Mode"=w201:u16, "Freq Mode"=w200:u16, "New Sampling Rate"=w199:dbl, "Use Default Name"=w198:bool, "x"=w197:bool, "y"=w196:bool, "z"=w195:bool, "All points"=w194:bool, "A_single val axis"=w193:u16, "B_single val axis"=w192:u16, "Use Default Value"=w191:bool, "Result Name"=w190:string, "Smoothing Width"=w189:i32, "Window"=w188:u16, "Para_dB"=w187:sgl, "Para_%"=w186:sgl, "Exponent"=w185:sgl, "Hz"=w184:u32, "Direct Weighting"=w183:bool, "Auto Inc"=w182:bool, "Inc(deg)"=w181:i32, "Total Rotation"=w180:i32, "Ref Freq Mode"=w179:u16, "Ref Waveform"=w178:string, "Sampling Rate"=w177:dbl, "Weighting Curve"=w176:string, "Ref Freq"=w175:dbl, "Curve Group"=w174:string[], "Search Items"=w173:string[], "Custom unit info"=w172:T7, "Unit"=w171:string, "Type A"=w170:enum16{"Curves", "Values", "Results", "WFM"}, "Type B"=w169:enum16{"Curves", "Values", "Results", "WFM"}, "Unary Operator"=w168:u16, "Binary Operator"=w167:u16, "Statistical Operator"=w166:u16, "New Resolution"=w165:u16, "Constant"=w164:dbl, "Help"=w160:string, "Tab Value"=w159:enum32{"Setting", "Help"}, "user equation cluster"=w158:T2)
              n37 = To Double Precision Float(number=w184) -> (double precision float=w162:dbl)
              n38 = Bundle By Name(cluster=w163, "Name"=w209, "Op Type"=w208, "Curve A"=w207, "Curve B"=w206, "Axis Mode"=w205, "Work Mode"=w204, "Width"=w203, "Weighting win"=w202, "Search Mode"=w201, "Freq Mode"=w200, "New Sampling Rate"=w199, "Use Default Name"=w198, "x"=w197, "y"=w196, "z"=w195, "All points"=w194, "A_single val axis"=w193, "B_single val axis"=w192, "Use Default Value"=w191, "Result Name"=w190, "Smoothing Width"=w189, "Window"=w188, "Para_dB"=w187, "Para_%"=w186, "Exponent"=w185, "Hz"=w162, "Direct Weighting"=w183, "Auto Inc"=w182, "Inc(deg)"=w181, "Total Rotation"=w180, "Ref Freq Mode"=w179, "Ref Waveform"=w178, "Sampling Rate"=w177, "Weighting Curve"=w176, "Ref Freq"=w175, "Curve Group"=w174, "Search Items"=w173, "Custom unit info"=w172, "Unit"=w171, "Type A"=w170, "Type B"=w169, "Unary Operator"=w168, "Binary Operator"=w167, "Statistical Operator"=w166, "New Resolution"=w165, "Constant"=w164, "Help"=w160, "Tab Value"=w159, "user equation cluster"=w158, "Work in Statics"=u16 0) -> (w210:T4)
            }
            frame 4 {
              w221 = T9 {"Name"="", "Op Type"=0, "Curve A"="", "Curve B"="", "Axis Mode"=0, "Work Mode"=0, "Width"=0, "Weighting win"=0, "Search Mode"=0, "Freq Mode"=0, "New Sampling Rate"=0.0, "Use Default Name"=FALSE, "x"=FALSE, "y"=FALSE, "z"=FALSE, "All points"=FALSE, "A_single val axis"=0, "B_single val axis"=0, "Use Default Value"=FALSE, "Result Name"="", "Smoothing Width"=0, "Window"=0, "Para_dB"=0.0, "Para_%"=0.0, "Exponent"=0.0, "Hz"=0.0, "Direct Weighting"=FALSE, "Auto Inc"=FALSE, "Inc(deg)"=0, "Total Rotation"=0, "Ref Freq Mode"=0, "Ref Waveform"="", "Sampling Rate"=0.0, "Weighting Curve"="", "Ref Freq"=0.0, "Curve Group"=[], "Search Items"=[], "Custom unit info"={"use custom"=FALSE, "lin/log"=0, "unit"="", "dB ref"=0.0, "common dB"=0}, "Unit"="", "Type A"=enum."Curves", "Type B"=enum."Curves", "Unary Operator"=0, "Binary Operator"=0, "Statistical Operator"=0, "Constant "=0.0, "New Resolution"=0, "user equation cluster"={"Custom unit input array"=[], "Custom unit results array "=[], "Desired Result Variables"=[], "Desired Result Names"=[], "Input Curve Names"=[], "Input Curve Variables"=[], "equation"="", "Input axis"=[], "Results axis"=[], "# input curves"=0, "# Desired result curves "=0, "Input Values"=[], "Result Values"=[]}, "Help"="", "Tab Value"=enum."Setting"}  # Post-Processing4
              n39 = Unflatten From String(type=w221, binary string=w277) -> (value=w274:T9, error out=w275:errorcluster)  [unwired: 1 in, 3 out]
              n40 = Unbundle(w275) -> ("status"=w276:bool)  [unwired: 2 out]
              n41 = case shown="True" w276 {
                tunnel: w276 -> [_ w278]
                frame False {
                }
                frame True {
                  n42 = local write "Error?"(w278) -> ()
                }
              }
              n43 = Unbundle By Name(w274) -> ("Name"=w272:string, "Op Type"=w271:u16, "Curve A"=w270:string, "Curve B"=w269:string, "Axis Mode"=w268:u16, "Work Mode"=w267:u16, "Width"=w266:u16, "Weighting win"=w265:u16, "Search Mode"=w264:u16, "Freq Mode"=w263:u16, "New Sampling Rate"=w262:dbl, "Use Default Name"=w261:bool, "x"=w260:bool, "y"=w259:bool, "z"=w258:bool, "All points"=w257:bool, "A_single val axis"=w256:u16, "B_single val axis"=w255:u16, "Use Default Value"=w254:bool, "Result Name"=w253:string, "Smoothing Width"=w252:i32, "Window"=w251:u16, "Para_dB"=w250:sgl, "Para_%"=w249:sgl, "Exponent"=w248:sgl, "Hz"=w247:dbl, "Direct Weighting"=w246:bool, "Auto Inc"=w245:bool, "Inc(deg)"=w244:i32, "Total Rotation"=w243:i32, "Ref Freq Mode"=w242:u16, "Ref Waveform"=w241:string, "Sampling Rate"=w240:dbl, "Weighting Curve"=w239:string, "Ref Freq"=w238:dbl, "Curve Group"=w237:string[], "Search Items"=w236:string[], "Custom unit info"=w235:T7, "Unit"=w234:string, "Type A"=w233:enum16{"Curves", "Values", "Results", "WFM"}, "Type B"=w232:enum16{"Curves", "Values", "Results", "WFM"}, "Unary Operator"=w231:u16, "Binary Operator"=w230:u16, "Statistical Operator"=w229:u16, "New Resolution"=w228:u16, "Constant"=w227:dbl, "Help"=w224:string, "Tab Value"=w223:enum32{"Setting", "Help"}, "user equation cluster"=w222:T2, "Help"=w220:string, "Tab Value"=w219:enum32{"Setting", "Help"})
              n44 = To Double Precision Float(number=w247) -> (double precision float=w225:dbl)
              n45 = Bundle By Name(cluster=w226, "Name"=w272, "Op Type"=w271, "Curve A"=w270, "Curve B"=w269, "Axis Mode"=w268, "Work Mode"=w267, "Width"=w266, "Weighting win"=w265, "Search Mode"=w264, "Freq Mode"=w263, "New Sampling Rate"=w262, "Use Default Name"=w261, "x"=w260, "y"=w259, "z"=w258, "All points"=w257, "A_single val axis"=w256, "B_single val axis"=w255, "Use Default Value"=w254, "Result Name"=w253, "Smoothing Width"=w252, "Window"=w251, "Para_dB"=w250, "Para_%"=w249, "Exponent"=w248, "Hz"=w225, "Direct Weighting"=w246, "Auto Inc"=w245, "Inc(deg)"=w244, "Total Rotation"=w243, "Ref Freq Mode"=w242, "Ref Waveform"=w241, "Sampling Rate"=w240, "Weighting Curve"=w239, "Ref Freq"=w238, "Curve Group"=w237, "Search Items"=w236, "Custom unit info"=w235, "Unit"=w234, "Type A"=w233, "Type B"=w232, "Unary Operator"=w231, "Binary Operator"=w230, "Statistical Operator"=w229, "New Resolution"=w228, "Constant"=w227, "Help"=w224, "Tab Value"=w223, "user equation cluster"=w222, "Help"=w220, "Tab Value"=w219, "Zwciker_X-axis"=u16 0, "Zwicker_spectrum"=FALSE, "Work in Statics"=u16 0) -> (w273:T4)
            }
            frame 5 {
              w285 = T10 {"Name"="", "Op Type"=0, "Curve A"="", "Curve B"="", "Axis Mode"=0, "Work Mode"=0, "Width"=0, "Weighting win"=0, "Search Mode"=0, "Freq Mode"=0, "New Sampling Rate"=0.0, "Use Default Name"=FALSE, "x"=FALSE, "y"=FALSE, "z"=FALSE, "All points"=FALSE, "A_single val axis"=0, "B_single val axis"=0, "Use Default Value"=FALSE, "Result Name"="", "Smoothing Width"=0, "Window"=0, "Para_dB"=0.0, "Para_%"=0.0, "Exponent"=0.0, "Hz"=0.0, "Direct Weighting"=FALSE, "Auto Inc"=FALSE, "Inc(deg)"=0, "Total Rotation"=0, "Ref Freq Mode"=0, "Ref Waveform"="", "Sampling Rate"=0.0, "Weighting Curve"="", "Ref Freq"=0.0, "Curve Group"=[], "Search Items"=[], "Custom unit info"={"use custom"=FALSE, "lin/log"=0, "unit"="", "dB ref"=0.0, "common dB"=0}, "Unit"="", "Type A"=enum."Curves", "Type B"=enum."Curves", "Unary Operator"=0, "Binary Operator"=0, "Statistical Operator"=0, "Constant "=0.0, "New Resolution"=0, "user equation cluster"={"Custom unit input array"=[], "Custom unit results array "=[], "Desired Result Variables"=[], "Desired Result Names"=[], "Input Curve Names"=[], "Input Curve Variables"=[], "equation"="", "Input axis"=[], "Results axis"=[], "# input curves"=0, "# Desired result curves "=0, "Input Values"=[], "Result Values"=[]}, "Help"="", "Tab Value"=enum."Setting", "Zwciker_X-axis"=0, "Zwicker_spectrum"=FALSE}  # Post-Processing5
              n46 = Unflatten From String(type=w285, binary string=w343) -> (value=w340:T10, error out=w341:errorcluster)  [unwired: 1 in, 3 out]
              n47 = Unbundle(w341) -> ("status"=w342:bool)  [unwired: 2 out]
              n48 = case shown="True" w342 {
                tunnel: w342 -> [_ w344]
                frame False {
                }
                frame True {
                  n49 = local write "Error?"(w344) -> ()
                }
              }
              n50 = Unbundle By Name(w340) -> ("Name"=w338:string, "Op Type"=w337:u16, "Curve A"=w336:string, "Curve B"=w335:string, "Axis Mode"=w334:u16, "Work Mode"=w333:u16, "Width"=w332:u16, "Weighting win"=w331:u16, "Search Mode"=w330:u16, "Freq Mode"=w329:u16, "New Sampling Rate"=w328:dbl, "Use Default Name"=w327:bool, "x"=w326:bool, "y"=w325:bool, "z"=w324:bool, "All points"=w323:bool, "A_single val axis"=w322:u16, "B_single val axis"=w321:u16, "Use Default Value"=w320:bool, "Result Name"=w319:string, "Smoothing Width"=w318:i32, "Window"=w317:u16, "Para_dB"=w316:sgl, "Para_%"=w315:sgl, "Exponent"=w314:sgl, "Hz"=w313:dbl, "Direct Weighting"=w312:bool, "Auto Inc"=w311:bool, "Inc(deg)"=w310:i32, "Total Rotation"=w309:i32, "Ref Freq Mode"=w308:u16, "Ref Waveform"=w307:string, "Sampling Rate"=w306:dbl, "Weighting Curve"=w305:string, "Ref Freq"=w304:dbl, "Curve Group"=w303:string[], "Search Items"=w302:string[], "Custom unit info"=w301:T7, "Unit"=w300:string, "Type A"=w299:enum16{"Curves", "Values", "Results", "WFM"}, "Type B"=w298:enum16{"Curves", "Values", "Results", "WFM"}, "Unary Operator"=w297:u16, "Binary Operator"=w296:u16, "Statistical Operator"=w295:u16, "New Resolution"=w294:u16, "Constant"=w293:dbl, "Help"=w290:string, "Tab Value"=w289:enum32{"Setting", "Help"}, "user equation cluster"=w288:T2, "Help"=w287:string, "Tab Value"=w286:enum32{"Setting", "Help"}, "Zwciker_X-axis"=w284:u16, "Zwicker_spectrum"=w283:bool)
              n51 = To Double Precision Float(number=w313) -> (double precision float=w291:dbl)
              n52 = Bundle By Name(cluster=w292, "Name"=w338, "Op Type"=w337, "Curve A"=w336, "Curve B"=w335, "Axis Mode"=w334, "Work Mode"=w333, "Width"=w332, "Weighting win"=w331, "Search Mode"=w330, "Freq Mode"=w329, "New Sampling Rate"=w328, "Use Default Name"=w327, "x"=w326, "y"=w325, "z"=w324, "All points"=w323, "A_single val axis"=w322, "B_single val axis"=w321, "Use Default Value"=w320, "Result Name"=w319, "Smoothing Width"=w318, "Window"=w317, "Para_dB"=w316, "Para_%"=w315, "Exponent"=w314, "Hz"=w291, "Direct Weighting"=w312, "Auto Inc"=w311, "Inc(deg)"=w310, "Total Rotation"=w309, "Ref Freq Mode"=w308, "Ref Waveform"=w307, "Sampling Rate"=w306, "Weighting Curve"=w305, "Ref Freq"=w304, "Curve Group"=w303, "Search Items"=w302, "Custom unit info"=w301, "Unit"=w300, "Type A"=w299, "Type B"=w298, "Unary Operator"=w297, "Binary Operator"=w296, "Statistical Operator"=w295, "New Resolution"=w294, "Constant"=w293, "Help"=w290, "Tab Value"=w289, "user equation cluster"=w288, "Help"=w287, "Tab Value"=w286, "Zwciker_X-axis"=w284, "Zwicker_spectrum"=w283, "Freq Sampling Mode"=u16 0, "Freq Sampling Rate"=0.0, "Smoothing"=FALSE, "Work in Statics"=u16 0) -> (w339:T4)
            }
            frame 6 {
              w348 = T11 {"Name"="", "Op Type"=0, "Curve A"="", "Curve B"="", "Axis Mode"=0, "Work Mode"=0, "Width"=0, "Weighting win"=0, "Search Mode"=0, "Freq Mode"=0, "New Sampling Rate"=0.0, "Use Default Name"=FALSE, "x"=FALSE, "y"=FALSE, "z"=FALSE, "All points"=FALSE, "A_single val axis"=0, "B_single val axis"=0, "Use Default Value"=FALSE, "Result Name"="", "Smoothing Width"=0, "Window"=0, "Para_dB"=0.0, "Para_%"=0.0, "Exponent"=0.0, "Hz"=0.0, "Direct Weighting"=FALSE, "Auto Inc"=FALSE, "Inc(deg)"=0, "Total Rotation"=0, "Ref Freq Mode"=0, "Ref Waveform"="", "Sampling Rate"=0.0, "Weighting Curve"="", "Ref Freq"=0.0, "Curve Group"=[], "Search Items"=[], "Custom unit info"={"use custom"=FALSE, "lin/log"=0, "unit"="", "dB ref"=0.0, "common dB"=0}, "Unit"="", "Type A"=enum."Curves", "Type B"=enum."Curves", "Unary Operator"=0, "Binary Operator"=0, "Statistical Operator"=0, "Constant "=0.0, "New Resolution"=0, "user equation cluster"={"Custom unit input array"=[], "Custom unit results array "=[], "Desired Result Variables"=[], "Desired Result Names"=[], "Input Curve Names"=[], "Input Curve Variables"=[], "equation"="", "Input axis"=[], "Results axis"=[], "# input curves"=0, "# Desired result curves "=0, "Input Values"=[], "Result Values"=[]}, "Help"="", "Tab Value"=enum."Setting", "Zwciker_X-axis"=0, "Zwicker_spectrum"=FALSE, "Freq Sampling Mode"=0, "Freq Sampling Rate"=0.0}  # Post-Processing6
              n53 = Unflatten From String(type=w348, binary string=w409) -> (value=w406:T11, error out=w407:errorcluster)  [unwired: 1 in, 3 out]
              n54 = Unbundle(w407) -> ("status"=w408:bool)  [unwired: 2 out]
              n55 = case shown="True" w408 {
                tunnel: w408 -> [_ w410]
                frame False {
                }
                frame True {
                  n56 = local write "Error?"(w410) -> ()
                }
              }
              n57 = Unbundle By Name(w406) -> ("Name"=w404:string, "Op Type"=w403:u16, "Curve A"=w402:string, "Curve B"=w401:string, "Axis Mode"=w400:u16, "Work Mode"=w399:u16, "Width"=w398:u16, "Weighting win"=w397:u16, "Search Mode"=w396:u16, "Freq Mode"=w395:u16, "New Sampling Rate"=w394:dbl, "Use Default Name"=w393:bool, "x"=w392:bool, "y"=w391:bool, "z"=w390:bool, "All points"=w389:bool, "A_single val axis"=w388:u16, "B_single val axis"=w387:u16, "Use Default Value"=w386:bool, "Result Name"=w385:string, "Smoothing Width"=w384:i32, "Window"=w383:u16, "Para_dB"=w382:sgl, "Para_%"=w381:sgl, "Exponent"=w380:sgl, "Hz"=w379:dbl, "Direct Weighting"=w378:bool, "Auto Inc"=w377:bool, "Inc(deg)"=w376:i32, "Total Rotation"=w375:i32, "Ref Freq Mode"=w374:u16, "Ref Waveform"=w373:string, "Sampling Rate"=w372:dbl, "Weighting Curve"=w371:string, "Ref Freq"=w370:dbl, "Curve Group"=w369:string[], "Search Items"=w368:string[], "Custom unit info"=w367:T7, "Unit"=w366:string, "Type A"=w365:enum16{"Curves", "Values", "Results", "WFM"}, "Type B"=w364:enum16{"Curves", "Values", "Results", "WFM"}, "Unary Operator"=w363:u16, "Binary Operator"=w362:u16, "Statistical Operator"=w361:u16, "New Resolution"=w360:u16, "Constant"=w359:dbl, "Help"=w356:string, "Tab Value"=w355:enum32{"Setting", "Help"}, "user equation cluster"=w354:T2, "Help"=w353:string, "Tab Value"=w352:enum32{"Setting", "Help"}, "Zwciker_X-axis"=w351:u16, "Zwicker_spectrum"=w350:bool, "Freq Sampling Mode"=w347:u16, "Freq Sampling Rate"=w346:dbl)
              n58 = To Double Precision Float(number=w379) -> (double precision float=w357:dbl)
              n59 = Bundle By Name(cluster=w358, "Name"=w404, "Op Type"=w403, "Curve A"=w402, "Curve B"=w401, "Axis Mode"=w400, "Work Mode"=w399, "Width"=w398, "Weighting win"=w397, "Search Mode"=w396, "Freq Mode"=w395, "New Sampling Rate"=w394, "Use Default Name"=w393, "x"=w392, "y"=w391, "z"=w390, "All points"=w389, "A_single val axis"=w388, "B_single val axis"=w387, "Use Default Value"=w386, "Result Name"=w385, "Smoothing Width"=w384, "Window"=w383, "Para_dB"=w382, "Para_%"=w381, "Exponent"=w380, "Hz"=w357, "Direct Weighting"=w378, "Auto Inc"=w377, "Inc(deg)"=w376, "Total Rotation"=w375, "Ref Freq Mode"=w374, "Ref Waveform"=w373, "Sampling Rate"=w372, "Weighting Curve"=w371, "Ref Freq"=w370, "Curve Group"=w369, "Search Items"=w368, "Custom unit info"=w367, "Unit"=w366, "Type A"=w365, "Type B"=w364, "Unary Operator"=w363, "Binary Operator"=w362, "Statistical Operator"=w361, "New Resolution"=w360, "Constant"=w359, "Help"=w356, "Tab Value"=w355, "user equation cluster"=w354, "Help"=w353, "Tab Value"=w352, "Zwciker_X-axis"=w351, "Zwicker_spectrum"=w350, "Freq Sampling Mode"=w347, "Freq Sampling Rate"=w346, "Smoothing"=FALSE, "Work in Statics"=u16 0) -> (w405:T4)
            }
            frame 7 {
              w412 = T12 {"Name"="", "Op Type"=0, "Curve A"="", "Curve B"="", "Axis Mode"=0, "Work Mode"=0, "Width"=0, "Weighting win"=0, "Search Mode"=0, "Freq Mode"=0, "New Sampling Rate"=0.0, "Use Default Name"=FALSE, "x"=FALSE, "y"=FALSE, "z"=FALSE, "All points"=FALSE, "A_single val axis"=0, "B_single val axis"=0, "Use Default Value"=FALSE, "Result Name"="", "Smoothing Width"=0, "Window"=0, "Para_dB"=0.0, "Para_%"=0.0, "Exponent"=0.0, "Hz"=0.0, "Direct Weighting"=FALSE, "Auto Inc"=FALSE, "Inc(deg)"=0, "Total Rotation"=0, "Ref Freq Mode"=0, "Ref Waveform"="", "Sampling Rate"=0.0, "Weighting Curve"="", "Ref Freq"=0.0, "Curve Group"=[], "Search Items"=[], "Custom unit info"={"use custom"=FALSE, "lin/log"=0, "unit"="", "dB ref"=0.0, "common dB"=0}, "Unit"="", "Type A"=enum."Curves", "Type B"=enum."Curves", "Unary Operator"=0, "Binary Operator"=0, "Statistical Operator"=0, "Constant "=0.0, "New Resolution"=0, "user equation cluster"={"Custom unit input array"=[], "Custom unit results array "=[], "Desired Result Variables"=[], "Desired Result Names"=[], "Input Curve Names"=[], "Input Curve Variables"=[], "equation"="", "Input axis"=[], "Results axis"=[], "# input curves"=0, "# Desired result curves "=0, "Input Values"=[], "Result Values"=[]}, "Help"="", "Tab Value"=enum."Setting", "Zwciker_X-axis"=0, "Zwicker_spectrum"=FALSE, "Freq Sampling Mode"=0, "Freq Sampling Rate"=0.0, "Smoothing"=FALSE}  # Post-Processing7
              n60 = Unflatten From String(type=w412, binary string=w475) -> (value=w472:T12, error out=w473:errorcluster)  [unwired: 1 in, 3 out]
              n61 = Unbundle(w473) -> ("status"=w474:bool)  [unwired: 2 out]
              n62 = case shown="True" w474 {
                tunnel: w474 -> [_ w476]
                frame False {
                }
                frame True {
                  n63 = local write "Error?"(w476) -> ()
                }
              }
              n64 = Unbundle By Name(w472) -> ("Name"=w470:string, "Op Type"=w469:u16, "Curve A"=w468:string, "Curve B"=w467:string, "Axis Mode"=w466:u16, "Work Mode"=w465:u16, "Width"=w464:u16, "Weighting win"=w463:u16, "Search Mode"=w462:u16, "Freq Mode"=w461:u16, "New Sampling Rate"=w460:dbl, "Use Default Name"=w459:bool, "x"=w458:bool, "y"=w457:bool, "z"=w456:bool, "All points"=w455:bool, "A_single val axis"=w454:u16, "B_single val axis"=w453:u16, "Use Default Value"=w452:bool, "Result Name"=w451:string, "Smoothing Width"=w450:i32, "Window"=w449:u16, "Para_dB"=w448:sgl, "Para_%"=w447:sgl, "Exponent"=w446:sgl, "Hz"=w445:dbl, "Direct Weighting"=w444:bool, "Auto Inc"=w443:bool, "Inc(deg)"=w442:i32, "Total Rotation"=w441:i32, "Ref Freq Mode"=w440:u16, "Ref Waveform"=w439:string, "Sampling Rate"=w438:dbl, "Weighting Curve"=w437:string, "Ref Freq"=w436:dbl, "Curve Group"=w435:string[], "Search Items"=w434:string[], "Custom unit info"=w433:T7, "Unit"=w432:string, "Type A"=w431:enum16{"Curves", "Values", "Results", "WFM"}, "Type B"=w430:enum16{"Curves", "Values", "Results", "WFM"}, "Unary Operator"=w429:u16, "Binary Operator"=w428:u16, "Statistical Operator"=w427:u16, "New Resolution"=w426:u16, "Constant"=w425:dbl, "Help"=w422:string, "Tab Value"=w421:enum32{"Setting", "Help"}, "user equation cluster"=w420:T2, "Help"=w419:string, "Tab Value"=w418:enum32{"Setting", "Help"}, "Zwciker_X-axis"=w417:u16, "Zwicker_spectrum"=w416:bool, "Freq Sampling Mode"=w414:u16, "Freq Sampling Rate"=w413:dbl)
              n65 = To Double Precision Float(number=w445) -> (double precision float=w423:dbl)
              n66 = Bundle By Name(cluster=w424, "Name"=w470, "Op Type"=w469, "Curve A"=w468, "Curve B"=w467, "Axis Mode"=w466, "Work Mode"=w465, "Width"=w464, "Weighting win"=w463, "Search Mode"=w462, "Freq Mode"=w461, "New Sampling Rate"=w460, "Use Default Name"=w459, "x"=w458, "y"=w457, "z"=w456, "All points"=w455, "A_single val axis"=w454, "B_single val axis"=w453, "Use Default Value"=w452, "Result Name"=w451, "Smoothing Width"=w450, "Window"=w449, "Para_dB"=w448, "Para_%"=w447, "Exponent"=w446, "Hz"=w423, "Direct Weighting"=w444, "Auto Inc"=w443, "Inc(deg)"=w442, "Total Rotation"=w441, "Ref Freq Mode"=w440, "Ref Waveform"=w439, "Sampling Rate"=w438, "Weighting Curve"=w437, "Ref Freq"=w436, "Curve Group"=w435, "Search Items"=w434, "Custom unit info"=w433, "Unit"=w432, "Type A"=w431, "Type B"=w430, "Unary Operator"=w429, "Binary Operator"=w428, "Statistical Operator"=w427, "New Resolution"=w426, "Constant"=w425, "Help"=w422, "Tab Value"=w421, "user equation cluster"=w420, "Help"=w419, "Tab Value"=w418, "Zwciker_X-axis"=w417, "Zwicker_spectrum"=w416, "Freq Sampling Mode"=w414, "Freq Sampling Rate"=w413, "Smoothing"=FALSE, "Work in Statics"=u16 0) -> (w471:T4)
            }
            frame 8 {
              w477 = T13 {"Name"="", "Op Type"=0, "Curve A"="", "Curve B"="", "Axis Mode"=0, "Work Mode"=0, "Width"=0, "Weighting win"=0, "Search Mode"=0, "Freq Mode"=0, "New Sampling Rate"=0.0, "Use Default Name"=FALSE, "x"=FALSE, "y"=FALSE, "z"=FALSE, "All points"=FALSE, "A_single val axis"=0, "B_single val axis"=0, "Use Default Value"=FALSE, "Result Name"="", "Smoothing Width"=0, "Window"=0, "Para_dB"=0.0, "Para_%"=0.0, "Exponent"=0.0, "Hz"=0.0, "Direct Weighting"=FALSE, "Auto Inc"=FALSE, "Inc(deg)"=0, "Total Rotation"=0, "Ref Freq Mode"=0, "Ref Waveform"="", "Sampling Rate"=0.0, "Weighting Curve"="", "Ref Freq"=0.0, "Curve Group"=[], "Search Items"=[], "Custom unit info"={"use custom"=FALSE, "lin/log"=0, "unit"="", "dB ref"=0.0, "common dB"=0}, "Unit"="", "Type A"=enum."Curves", "Type B"=enum."Curves", "Unary Operator"=0, "Binary Operator"=0, "Statistical Operator"=0, "Constant "=0.0, "New Resolution"=0, "user equation cluster"={"Custom unit input array"=[], "Custom unit results array "=[], "Desired Result Variables"=[], "Desired Result Names"=[], "Input Curve Names"=[], "Input Curve Variables"=[], "equation"="", "Input axis"=[], "Results axis"=[], "# input curves"=0, "# Desired result curves "=0, "Input Values"=[], "Result Values"=[]}, "Help"="", "Tab Value"=enum."Setting", "Zwciker_X-axis"=0, "Zwicker_spectrum"=FALSE, "Freq Sampling Mode"=0, "Freq Sampling Rate"=0.0, "Smoothing"=FALSE, "Work in Statics"=0}  # Post-Processing8
              n67 = Unflatten From String(type=w477, binary string=w541) -> (value=w538:T13, error out=w539:errorcluster)  [unwired: 1 in, 3 out]
              n68 = Unbundle(w539) -> ("status"=w540:bool)  [unwired: 2 out]
              n69 = case shown="True" w540 {
                tunnel: w540 -> [_ w542]
                frame False {
                }
                frame True {
                  n70 = local write "Error?"(w542) -> ()
                }
              }
              n71 = Unbundle By Name(w538) -> ("Name"=w536:string, "Op Type"=w535:u16, "Curve A"=w534:string, "Curve B"=w533:string, "Axis Mode"=w532:u16, "Work Mode"=w531:u16, "Width"=w530:u16, "Weighting win"=w529:u16, "Search Mode"=w528:u16, "Freq Mode"=w527:u16, "New Sampling Rate"=w526:dbl, "Use Default Name"=w525:bool, "x"=w524:bool, "y"=w523:bool, "z"=w522:bool, "All points"=w521:bool, "A_single val axis"=w520:u16, "B_single val axis"=w519:u16, "Use Default Value"=w518:bool, "Result Name"=w517:string, "Smoothing Width"=w516:i32, "Window"=w515:u16, "Para_dB"=w514:sgl, "Para_%"=w513:sgl, "Exponent"=w512:sgl, "Hz"=w511:dbl, "Direct Weighting"=w510:bool, "Auto Inc"=w509:bool, "Inc(deg)"=w508:i32, "Total Rotation"=w507:i32, "Ref Freq Mode"=w506:u16, "Ref Waveform"=w505:string, "Sampling Rate"=w504:dbl, "Weighting Curve"=w503:string, "Ref Freq"=w502:dbl, "Curve Group"=w501:string[], "Search Items"=w500:string[], "Custom unit info"=w499:T7, "Unit"=w498:string, "Type A"=w497:enum16{"Curves", "Values", "Results", "WFM"}, "Type B"=w496:enum16{"Curves", "Values", "Results", "WFM"}, "Unary Operator"=w495:u16, "Binary Operator"=w494:u16, "Statistical Operator"=w493:u16, "New Resolution"=w492:u16, "Constant"=w491:dbl, "Help"=w488:string, "Tab Value"=w487:enum32{"Setting", "Help"}, "user equation cluster"=w486:T2, "Help"=w485:string, "Tab Value"=w484:enum32{"Setting", "Help"}, "Zwciker_X-axis"=w483:u16, "Zwicker_spectrum"=w482:bool, "Freq Sampling Mode"=w480:u16, "Freq Sampling Rate"=w479:dbl)
              n72 = To Double Precision Float(number=w511) -> (double precision float=w489:dbl)
              n73 = Bundle By Name(cluster=w490, "Name"=w536, "Op Type"=w535, "Curve A"=w534, "Curve B"=w533, "Axis Mode"=w532, "Work Mode"=w531, "Width"=w530, "Weighting win"=w529, "Search Mode"=w528, "Freq Mode"=w527, "New Sampling Rate"=w526, "Use Default Name"=w525, "x"=w524, "y"=w523, "z"=w522, "All points"=w521, "A_single val axis"=w520, "B_single val axis"=w519, "Use Default Value"=w518, "Result Name"=w517, "Smoothing Width"=w516, "Window"=w515, "Para_dB"=w514, "Para_%"=w513, "Exponent"=w512, "Hz"=w489, "Direct Weighting"=w510, "Auto Inc"=w509, "Inc(deg)"=w508, "Total Rotation"=w507, "Ref Freq Mode"=w506, "Ref Waveform"=w505, "Sampling Rate"=w504, "Weighting Curve"=w503, "Ref Freq"=w502, "Curve Group"=w501, "Search Items"=w500, "Custom unit info"=w499, "Unit"=w498, "Type A"=w497, "Type B"=w496, "Unary Operator"=w495, "Binary Operator"=w494, "Statistical Operator"=w493, "New Resolution"=w492, "Constant"=w491, "Help"=w488, "Tab Value"=w487, "user equation cluster"=w486, "Help"=w485, "Tab Value"=w484, "Zwciker_X-axis"=w483, "Zwicker_spectrum"=w482, "Freq Sampling Mode"=w480, "Freq Sampling Rate"=w479, "Smoothing"=FALSE, "Work in Statics"=u16 0) -> (w537:T4)
            }
            frame 9, Default {
              n74 = Unflatten From String(type=w543, binary string=w545) -> (value=w544:T4, error out=w546:errorcluster)  [unwired: 1 in, 3 out]
              n75 = Unbundle(w546) -> ("status"=w547:bool)  [unwired: 2 out]
              n76 = case shown="True" w547 {
                tunnel: w547 -> [_ w548]
                frame False {
                }
                frame True {
                  n77 = local write "Error?"(w548) -> ()
                }
              }
            }
          }
        }
      }
    }
    frame True {
      n78 = local write "Error?"(TRUE ("Error?")) -> ()
    }
  }
  "Post-Processing" <- w1
  n79 = Bundle("substring"=w5, w6, "unsigned byte array[2]"=w7) -> (→"Header info":T14)  [unwired: 1 out]
